vi "Scripted Autonomous.vi"   [LabVIEW 2015]
uses:
  Common Code/Change Detect Int.vi
  Robot Global Data.vi
types:
  T1 = typedef "Dashboard Control Data.ctl" = cluster{"Encoder Control":T2, "Steer PID output":cluster{"output high":dbl, "output low":dbl}, " Steer PID gains":cluster{"proportional gain (Kc)":dbl, "integral time (Ti, min)":dbl, "derivative time (Td, min)":dbl}, "Drivetrain Settings":T3, "Vision Packet":T4, "Dashboard Drivetrain Command":T5, "Info/Command Cluster":T7, "Ball Vision Packet":T8, "Intake Presets":T10, "Intake Encoder Control":T12, "Goal Output Range":cluster{"output high":dbl, "output low":dbl}, "Enabled Systems":T13, "Auton Presets":T14, "Pressure M":dbl, "Pressure B":dbl, "Vision Timeout":dbl, "Auto-Shift":T15, "Catapult Setpoints":T16, "Climb Presets":T17}
  T2 = typedef "Encoder Control.ctl" = cluster{"Right Tick Constant":dbl, "Left Tick Constant":dbl, "Reset?":bool, "Y Dist":cluster{"PID gains":cluster{"proportional gain (Kc)":dbl, "integral time (Ti, min)":dbl, "derivative time (Td, min)":dbl}}, "Y Stop Thresh":dbl, "Y Stop Speed":dbl}
  T3 = typedef "Drivetrain Settings.ctl" = cluster{"Gyro Tolerance":dbl, "Throttle Ramp (ms)":dbl, "Kv":dbl, "Ka":dbl, "Feed Forward P":dbl, "Feed Forward D":dbl, "Goal Vision PID gains":cluster{"proportional gain (Kc)":dbl, "integral time (Ti, min)":dbl, "derivative time (Td, min)":dbl}, "Goal Detection Window":dbl, "Creep Rate":dbl, "Vision Throttle Threshold":dbl, "Min Turn Output":dbl, "Left Batter Angle":dbl, "Right Batter Angle":dbl}
  T4 = typedef "Goal Vision Packet.ctl" = cluster{"Distance":dbl, "Center X":dbl, "Center Y":dbl, "Found Target?":bool, "Robot Center":dbl, "Angle":dbl}
  T5 = typedef "Dashboard Drivetrain Command.ctl" = cluster{"Drivetrain Vision":T6}
  T6 = typedef "Drivetrain Vision.ctl" = cluster{"Goal Window":dbl, "Ball Window":dbl}
  T7 = typedef "Ball Tracking Command Cluster.ctl" = cluster{"Distance to Ball":dbl, "Desired Angle":dbl, "Command":enum16{"Turn to Ball", "Turn to Angle", "Get Distance"}, "Pixels from Center":dbl}
  T8 = typedef "Ball Vision Packet.ctl" = cluster{"Ball Detected?":bool, "Distance to Ball":dbl, "Desired Angle":dbl, "Pixels from Center":dbl, "Tracking mode":T9}
  T9 = typedef "Tracking Mode.ctl" = enum16{"Turn to Ball", "Turn to Angle"}
  T10 = typedef "Intake Presets.ctl" = cluster{"Intake Speed":dbl, "Outake Speed":dbl, "Angle Speed":dbl, "Angle Tolerance":dbl, "Encoder Scale":dbl, "Load Height":dbl, "Output Range":T11, "MaxCurrent":dbl, "Idle Height":dbl, "Max Height":dbl, "Reset Encoders?":bool, "PID gains":cluster{"proportional gain (Kc)":dbl, "integral time (Ti, min)":dbl, "derivative time (Td, min)":dbl}, "Drop Low Height ":dbl, "Rotation Power Max/Min":dbl, "Reset Delay":dbl, "Current Trip Delay":dbl}
  T11 = typedef "Drivetrain Output Range.ctl" = cluster{"output high":dbl, "output low":dbl}
  T12 = typedef "IntakeEcoderControl.ctl" = cluster{"Arm Tick Constant":dbl, "Reset?":bool, "Y Dist":cluster{"PID gains":cluster{"proportional gain (Kc)":dbl, "integral time (Ti, min)":dbl, "derivative time (Td, min)":dbl}}, "Y Stop Thresh":dbl, "Y Stop Speed":dbl}
  T13 = typedef "Enabled Systems.ctl" = cluster{"Shoot":bool, "Intake":bool, "DT":bool, "Gyro":bool, "100ms":bool, "US":bool}
  T14 = typedef "Autonomous Presets.ctl" = cluster{"Pitch Limit":dbl, "Roll Limit":dbl, "Start Position":dbl, "Cross Position":dbl}
  T15 = typedef "Auto Shift Cluster.ctl" = cluster{"Delay":dbl, "Speed Thresh":dbl, "Upshift Accel":dbl, "Upshift Throttle":dbl, "Upshift Throttle Accel":dbl, "Downshift Throttle":dbl, "Downshift Throttle Accel":dbl, "Pressure Threshold":dbl}
  T16 = typedef "Catapult Presets.ctl" = cluster{"Intake Danger Height":dbl, "Ball Security Delay ":dbl, "High PSI Minimum":dbl, "Shot Finish Delay":dbl, "Low PSI Minimum":dbl, "Idle Ball Security Wait ":dbl}
  T17 = typedef "Climb Presets.ctl" = cluster{"Winch Speed":dbl, "Wait until Fire":dbl, "Wait until Winch":dbl, "Wait until Stop":dbl}
  T18 = typedef "Auton Command Cluster.ctl" = cluster{"Command ID":i32, "maxTime":dbl, "Y Distance":dbl, "Heading":dbl, "Throttle":dbl, "Async":dbl, "Velocity":dbl, "Acceleration":dbl, "To":dbl, "Condition":dbl, "Shot Type":dbl, "Left RPM":dbl, "Override RPM":i32, "Override Angle":i32, "Right RPM":dbl, "Angle":dbl, "Intake Mode":i32, "Intake Cmd":i32, "Intake O":i32, "Eject O":i32, "Angle O":i32, "Arm O":i32, "Intake Speed":dbl, "Eject Speed":dbl, "Arm Angle":dbl, "Arm Speed":dbl, "Intake?":i32, "Eject?":i32, "Left":dbl, "Right":dbl, "Pivot Speed":dbl, "Y Dist":dbl, "Position":dbl, "Desired Position":i32, "Shooter Mode":dbl, "Shooter Command":dbl, "Shoot?":i32, "Shoot mode":i32, "High Pressure?":i32, "Override IR ID ":i32}
  T19 = typedef "Drivetrain Status Cluster.ctl" = cluster{"Modes":T20, "Y (Throttle)":dbl, "X (Steer)":dbl, "Gyro In Range?":bool, "Distance Drive Finished?":bool, "Stop Eject Lockout":bool, "Dist Drive Status":T21, "Y Target":dbl, "Heading Target":dbl, "Vision Target Aligned?":bool}
  T20 = typedef "Drivetrain Modes.ctl" = enum16{"Gyro Steer", "Manual", "Goal Vision Targeting", "PID Distance Drive", "Hybrid"}
  T21 = typedef "Dist Drive Status.ctl" = cluster{"Y In Range":bool, "X In Range":bool, "Gyro In Range":bool, "Y Dist":dbl, "X Dist":dbl, "Gyro":dbl}
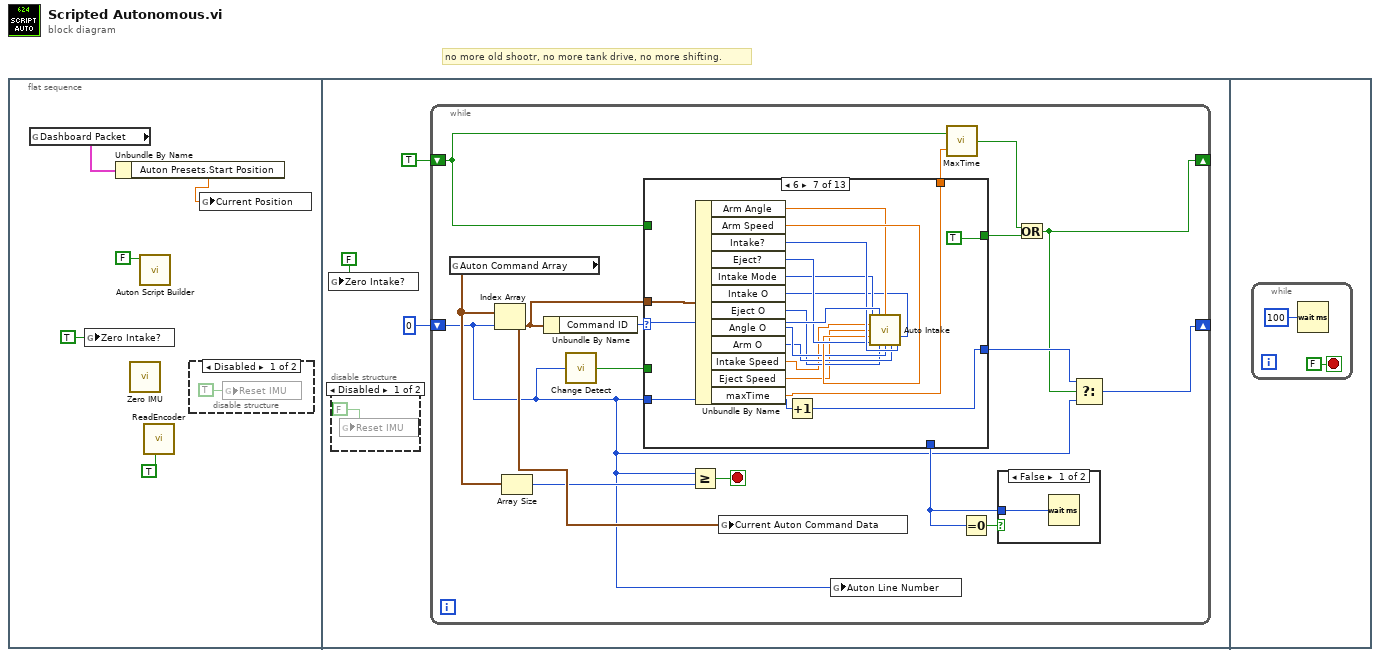
[diagram p0: block diagram]
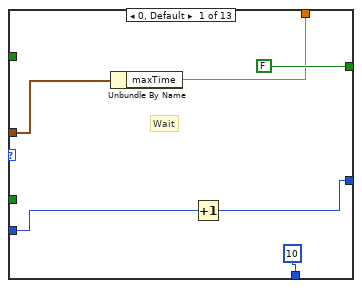
[diagram p5: hidden frame]
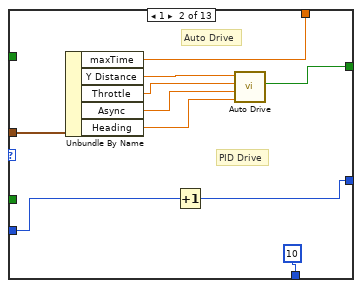
[diagram p6: hidden frame]
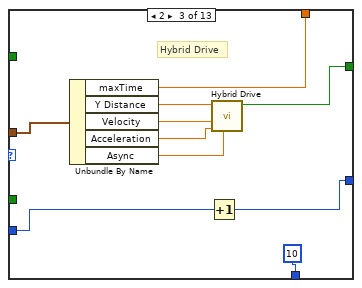
[diagram p7: hidden frame]
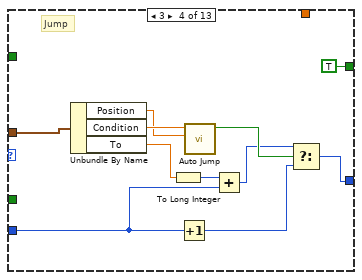
[diagram p8: hidden frame]
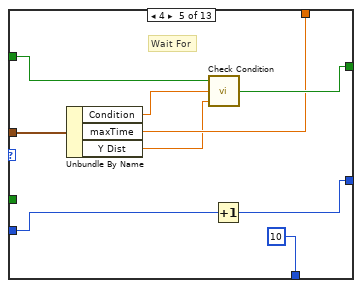
[diagram p9: hidden frame]
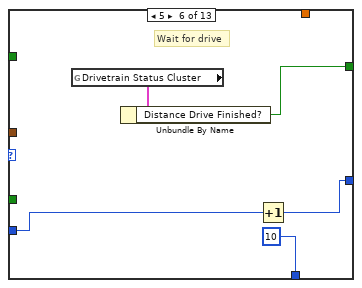
[diagram p10: hidden frame]
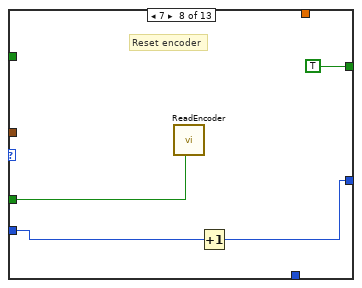
[diagram p11: hidden frame]
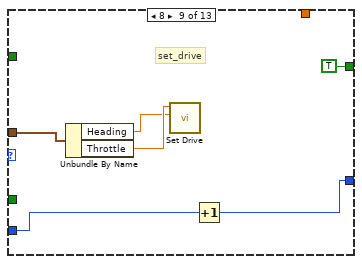
[diagram p12: hidden frame]
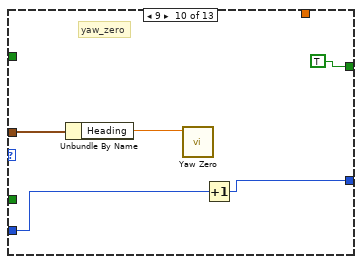
[diagram p13: hidden frame]
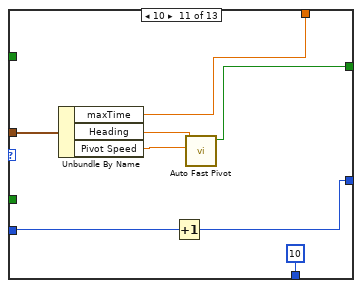
[diagram p14: hidden frame]
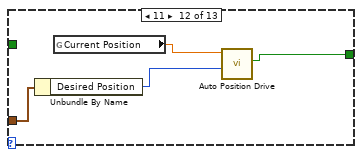
[diagram p15: hidden frame]
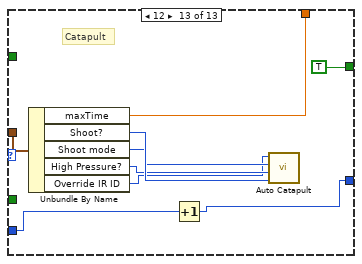
[diagram p16: hidden frame]
diagram:
  # "no more old shootr, no more tank drive, no more shifting."
  n1 = flat-sequence {
    frame #0 {
      n2 = global read "Robot Global Data.vi" "Dashboard Packet"() -> (w2:T1)
      n3 = global write "Robot Global Data.vi" "Zero Intake?"(TRUE ("Zero Intake?")) -> ()
      n4 = Unbundle By Name(w2) -> ("Auton Presets.Start Position"=w1:dbl)
      n5 = call "Zero IMU.vi"() -> ()  [unwired: 12 in]
      n6 = call "Auton Script Builder.vi"("Export?"=FALSE) -> ()  [unwired: 11 in]
      n7 = call "ReadEncoder.vi"("Reset?"=TRUE) -> ()  [unwired: 10 in, 1 out]
      n8 = disable-structure shown="Disabled" {
        frame Disabled {
          n9 = global write "Robot Global Data.vi" "Reset IMU"(TRUE ("Reset IMU")) -> ()
        }
        frame Enabled {
        }
      }
      n10 = global write "Robot Global Data.vi" "Current Position"(w1) -> ()
    }
    frame #1 {
      n11 = global write "Robot Global Data.vi" "Zero Intake?"(FALSE ("Zero Intake?")) -> ()
      n12 = disable-structure shown="Disabled" {
        frame Disabled {
          n13 = global write "Robot Global Data.vi" "Reset IMU"(FALSE ("Reset IMU")) -> ()
        }
        frame Enabled {
        }
      }
      n14 = while {
        shift-right: [w20] -> _
        shift-left: 0 -> [w11]
        shift-right: [w17] -> _
        shift-left: TRUE -> [w14]
        stop <- w21 stop-if-true
        n15 = global read "Robot Global Data.vi" "Auton Command Array"() -> (w23:T18[])
        n16 = Index Array(array=w23, index=w11) -> (element=w26:T18)
        n17 = Array Size(array=w23) -> (size(s)=w22:i32)
        n18 = Unbundle By Name(w26) -> ("Command ID"=w25:i32)
        n19 = call-poly "Change Detect.vi"("In"=w11) -> ("Changed?"=w24:bool)
        n20 = case shown="6" w25 {
          selector: w25 -> [_ _ _ _ _ _ w95 _ _ _ _ _ _]
          tunnel: w11 -> [w31 w36 w46 w59 w67 w77 w82 w97 w103 w109 w113 _ w130]
          tunnel: w24 -> [_ _ _ _ _ _ _ w99 _ _ _ _ _]
          tunnel: w14 -> [_ _ _ _ w73 _ _ _ _ _ _ _ _]
          tunnel: [w32 w35 w45 w55 w65 w78 w81 w96 w102 w108 w112 _ w129] -> w19
          tunnel: [FALSE w37 w49 TRUE ("Distance Drive Finished?") w72 w76 TRUE TRUE ("Distance Drive Finished?") TRUE ("Distance Drive Finished?") TRUE w115 w119 TRUE] -> w18
          tunnel: [w29 w42 w47 _ w70 _ w79 _ _ _ w114 _ w128] -> w15
          tunnel: w26 -> [w30 w43 w53 w63 w68 _ w94 _ w105 w107 w118 w122 w131]
          tunnel: [10 10 10 _ 10 10 _ _ _ _ 10 _ _] -> w13
          frame 0, Default {
            # "Wait"
            n21 = Unbundle By Name(w30) -> ("maxTime"=w29:dbl)
            n22 = Increment(x=w31) -> (x+1=w32:i32)
          }
          frame 1 {
            # "Auto Drive"
            # "PID Drive"
            n23 = Unbundle By Name(w43) -> ("maxTime"=w42:dbl, "Y Distance"=w41:dbl, "Throttle"=w40:dbl, "Async"=w39:dbl, "Heading"=w38:dbl)
            n24 = Increment(x=w36) -> (x+1=w35:i32)
            n25 = call "Auto Drive.vi"("heading"=w38, "async"=w39, "speed"=w40, "y"=w41) -> ("isFinished?"=w37:bool)  [unwired: 7 in]
          }
          frame 2 {
            # "Hybrid Drive"
            n26 = Unbundle By Name(w53) -> ("maxTime"=w47:dbl, "Y Distance"=w52:dbl, "Velocity"=w51:dbl, "Acceleration"=w50:dbl, "Async"=w48:dbl)
            n27 = Increment(x=w46) -> (x+1=w45:i32)
            n28 = call "Hybrid Drive.vi"("Async?"=w48, "Max Accel"=w50, "Max Velocity"=w51, "Distance"=w52) -> ("Finished?"=w49:bool)  [unwired: 7 in]
          }
          frame 3 {
            # "Jump"
            n29 = Unbundle By Name(w63) -> ("Position"=w54:dbl, "Condition"=w62:dbl, "To"=w57:dbl)
            n30 = To Long Integer(number=w57) -> (32bit integer=w58:i32)
            n31 = Increment(x=w59) -> (x+1=w60:i32)
            n32 = call "Auto Jump.vi"("Position"=w54, "Condition"=w62) -> ("Jump?"=w61:bool)  [unwired: 9 in]
            n33 = Add(x=w58, y=w59) -> (x+y=w56:i32)
            n34 = Select(t=w56, s=w61, f=w60) -> (s? t:f=w55:i32)
          }
          frame 4 {
            # "Wait For"
            n35 = Unbundle By Name(w68) -> ("Condition"=w71:dbl, "maxTime"=w70:dbl, "Y Dist"=w69:dbl)
            n36 = call "Check Condition.vi"("Distance"=w69, "Condition"=w71, "Reset"=w73) -> ("Done"=w72:bool)
            n37 = Increment(x=w67) -> (x+1=w65:i32)
          }
          frame 5 {
            # "Wait for drive"
            n38 = global read "Robot Global Data.vi" "Drivetrain Status Cluster"() -> (w75:T19)
            n39 = Unbundle By Name(w75) -> ("Distance Drive Finished?"=w76:bool)
            n40 = Increment(x=w77) -> (x+1=w78:i32)
          }
          frame 6 {
            n41 = Unbundle By Name(w94) -> ("Arm Angle"=w90:dbl, "Arm Speed"=w91:dbl, "Intake?"=w93:i32, "Eject?"=w92:i32, "Intake Mode"=w89:i32, "Intake O"=w85:i32, "Eject O"=w86:i32, "Angle O"=w88:i32, "Arm O"=w87:i32, "Intake Speed"=w83:dbl, "Eject Speed"=w84:dbl, "maxTime"=w79:dbl)
            n42 = Increment(x=w82) -> (x+1=w81:i32)
            n43 = call "Auto Intake.vi"("Intake Mode ID"=w89, "Intake Command ID"=w95, "Arm Angle"=w90, "Intake Override Speed"=w83, "Eject Override Speed"=w84, "Arm Speed"=w91, "Override Intake?"=w85, "Intake?"=w92, "Override Eject?"=w86, "Override Angle?"=w88, "Override Arm?"=w87, "Eject?"=w93) -> ()  [unwired: 4 in]
          }
          frame 7 {
            # "Reset encoder"
            n44 = call "ReadEncoder.vi"("Reset?"=w99) -> ()  [unwired: 10 in, 1 out]
            n45 = Increment(x=w97) -> (x+1=w96:i32)
          }
          frame 8 {
            # "set_drive"
            n46 = Unbundle By Name(w105) -> ("Heading"=w100:dbl, "Throttle"=w101:dbl)
            n47 = call "Set Drive.vi"("Heading Target"=w100, "Y Power"=w101) -> ()  [unwired: 10 in]
            n48 = Increment(x=w103) -> (x+1=w102:i32)
          }
          frame 9 {
            # "yaw_zero"
            n49 = Unbundle By Name(w107) -> ("Heading"=w106:dbl)
            n50 = call "Yaw Zero.vi"("Angle"=w106) -> ()  [unwired: 11 in]
            n51 = Increment(x=w109) -> (x+1=w108:i32)
          }
          frame 10 {
            n52 = Unbundle By Name(w118) -> ("maxTime"=w114:dbl, "Heading"=w116:dbl, "Pivot Speed"=w117:dbl)
            n53 = Increment(x=w113) -> (x+1=w112:i32)
            n54 = call "Auto Fast Pivot.vi"("Pivot Speed"=w117, "Heading"=w116) -> ("Done?"=w115:bool)  [unwired: 9 in]
          }
          frame 11 {
            n55 = Unbundle By Name(w122) -> ("Desired Position"=w120:i32)
            n56 = global read "Robot Global Data.vi" "Current Position"() -> (w121:dbl)
            n57 = call "Auto Position Drive.vi"("Desired Position"=w120, "Current Position"=w121) -> ("Finished?"=w119:bool)  [unwired: 9 in]
          }
          frame 12 {
            # "Catapult"
            n58 = Unbundle By Name(w131) -> ("maxTime"=w128:dbl, "Shoot?"=w127:i32, "Shoot mode"=w126:i32, "High Pressure?"=w125:i32, "Override IR ID"=w124:i32)
            n59 = Increment(x=w130) -> (x+1=w129:i32)
            n60 = call "Auto Catapult.vi"("Shoot ID"=w127, "High Pressure ID"=w125, "Shoot Mode ID"=w126, "Override IR ID"=w124) -> ()  [unwired: 7 in, 1 out]
          }
        }
        n61 = Greater Or Equal?(x=w11, y=w22) -> (x >= y?=w21:bool)
        n62 = global write "Robot Global Data.vi" "Current Auton Command Data"(w26) -> ()
        n63 = global write "Robot Global Data.vi" "Auton Line Number"(w11) -> ()
        n64 = call "MaxTime.vi"("MaxTime"=w15, "Reset?"=w14) -> ("Finished?"=w16:bool)
        n65 = Equal To 0?(x=w13) -> (x = 0?=w12:bool)
        n66 = case shown="False" w12 {
          tunnel: w13 -> [w27 _]
          frame False {
            n67 = Wait (ms)(milliseconds to wait=w27) -> ()  [unwired: 1 out]
          }
          frame True {
          }
        }
        n68 = Or(x=w16, y=w18) -> (x .or. y?=w17:bool)
        n69 = Select(t=w19, s=w17, f=w11) -> (s? t:f=w20:i32)
      }
    }
    frame #2 {
      n70 = while {
        stop <- FALSE stop-if-true
        n71 = Wait (ms)(milliseconds to wait=u32 100) -> ()  [unwired: 1 out]
      }
    }
  }
